vi "ToString.vi"(8 "error in (no error)":errorcluster, 11 "xmlNode in":refnum<class "xmlNode.lvclass">) -> (0 "error out":errorcluster, 2 "xml":string, 3 "xmlNode out":refnum<class "xmlNode.lvclass">)   [LabVIEW 2009, in "Tools.lvlib" / "xml.lvlib" / "xmlNode.lvclass"]
doc: "xml node to xml string (omits the xml title string at the head of an xml document)."
uses:
  xmlNode.lvclass
  xmlNode.lvclass/xmlNode.ctl
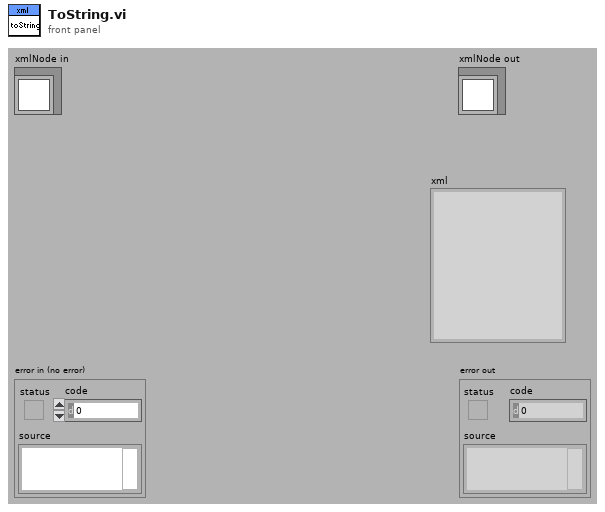
[diagram p1: front panel]
types:
  T1 = cluster{"attribute type":string, "attribute string":string}[]
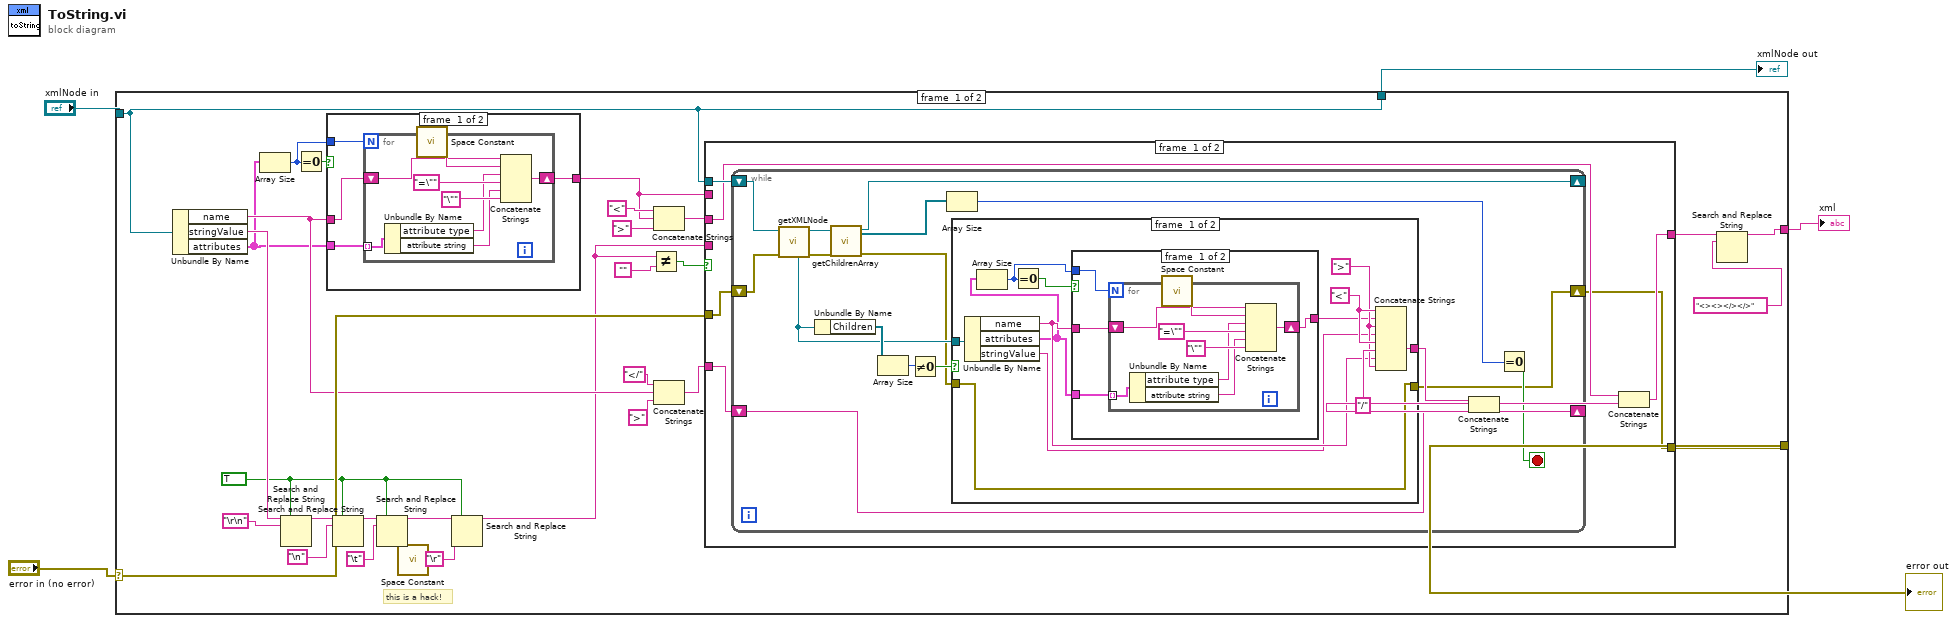
[diagram p0: block diagram]
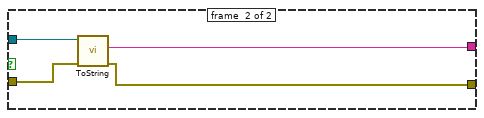
[diagram p4: hidden frame]
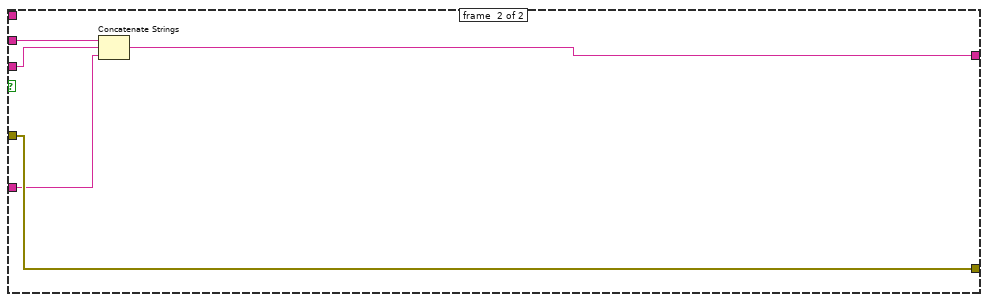
[diagram p5: hidden frame]
diagram:
  n1 = case shown="No Error" "error in (no error)" {
    selector: "error in (no error)" -> [w34 w107]
    tunnel: [w27 w107] -> w4
    tunnel: [w19 w106] -> w2
    tunnel: "xmlNode in" -> [w19 w106]
    tunnel: [w15 _] -> w1
    frame #0 {
      w11 = TRUE
      # "this is a hack!"
      n2 = Unbundle By Name(w19) -> ("name"=w17:string, "stringValue"=w22:string, "attributes"=w6:T1)
      n3 = Array Size(array=w6) -> (size(s)=w7:i32)
      n4 = Search and Replace String(replace all?=w11, input string=w22, search string="\r\n") -> (result string=w26:string)  [unwired: 5 in, 3 out]
      n5 = Equal To 0?(x=w7) -> (x = 0?=w8:bool)
      n6 = case shown="False" w8 {
        tunnel: [w38 w47] -> w18
        tunnel: w17 -> [w37 w47]
        tunnel: w7 -> [w36 _]
        tunnel: w6 -> [w35 _]
        frame #0 {
          n7 = for {
            N: w36 -> [_]
            shift-right: [w43] -> w38
            shift-left: w37 -> [w42]
            tunnel: w35 -> [w41] mode=indexing
            n8 = Unbundle By Name(w41) -> ("attribute type"=w40:string, "attribute string"=w39:string)
            n9 = call <vilib>:"Space Constant.vi"() -> ("String"=w46:string)
            n10 = Concatenate Strings(w42, w46, w40, "=\"", w39, "\"") -> (w43:string)
          }
        }
        frame #1 {
        }
      }
      n11 = Search and Replace String(replace all?=w11, input string=w26, search string="\n") -> (result string=w24:string)  [unwired: 5 in, 3 out]
      n12 = Search and Replace String(replace all?=w11, input string=w24, search string="\t") -> (result string=w9:string)  [unwired: 5 in, 3 out]
      n13 = call <vilib>:"Space Constant.vi"() -> ()  [unwired: 1 out]
      n14 = Search and Replace String(replace all?=w11, input string=w9, search string="\r") -> (result string=w13:string)  [unwired: 5 in, 3 out]
      n15 = Not Equal?(x=w13, y="") -> (x != y?=w12:bool)
      n16 = Concatenate Strings("<", w18, ">") -> (w31:string)
      n17 = Concatenate Strings("</", w17, ">") -> (w28:string)
      n18 = case shown="False" w12 {
        tunnel: w34 -> [w50 w102]
        tunnel: w13 -> [_ w104]
        tunnel: w31 -> [w52 w105]
        tunnel: w18 -> [_ _]
        tunnel: [w51 w103] -> w16
        tunnel: w19 -> [w54 _]
        tunnel: w28 -> [w48 w101]
        tunnel: [w49 w102] -> w27
        frame #0 {
          n19 = while {
            shift-right: [w68] -> _
            shift-left: w54 -> [w65]
            shift-right: [w57] -> w49
            shift-left: w50 -> [w56]
            shift-right: [w58] -> w53
            shift-left: w48 -> [w55]
            stop <- w70 stop-if-true
            n20 = call-dynamic "getXMLNode.vi"("error in (no error)"=w56, "xmlNode in"=w65) -> ("error out"=w66:errorcluster, "xmlNode extracted"=w61:refnum<class "xmlNode.lvclass">, "xmlNode out"=w67:refnum<class "xmlNode.lvclass">)  [unwired: 7 in]
            n21 = Unbundle By Name(w61) -> ("Children"=w64:refnum<class>[])
            n22 = call-dynamic "getChildrenArray.vi"("error in (no error)"=w66, "xmlNode.lvclass in"=w67) -> ("error out"=w60:errorcluster, "Children"=w71:refnum<class "xmlNode.lvclass">[], "xmlNode.lvclass out"=w68:refnum<class "xmlNode.lvclass">)  [unwired: 7 in]
            n23 = Array Size(array=w64) -> (size(s)=w63:i32)
            n24 = Not Equal To 0?(x=w63) -> (x != 0?=w62:bool)
            n25 = Array Size(array=w71) -> (size(s)=w69:i32)
            n26 = case shown="False" w62 {
              tunnel: w61 -> [w83 w100]
              tunnel: w60 -> [w82 w99]
              tunnel: [w78 w98] -> w59
              tunnel: [w82 w97] -> w57
              frame #0 {
                w79 = ">"
                w81 = "<"
                n27 = Unbundle By Name(w83) -> ("name"=w76:string, "attributes"=w73:T1, "stringValue"=w75:string)
                n28 = Array Size(array=w73) -> (size(s)=w72:i32)
                n29 = Equal To 0?(x=w72) -> (x = 0?=w74:bool)
                n30 = case shown="False" w74 {
                  tunnel: [w87 w96] -> w77
                  tunnel: w76 -> [w86 w96]
                  tunnel: w72 -> [w85 _]
                  tunnel: w73 -> [w84 _]
                  frame #0 {
                    n31 = for {
                      N: w85 -> [_]
                      shift-right: [w92] -> w87
                      shift-left: w86 -> [w91]
                      tunnel: w84 -> [w90] mode=indexing
                      n32 = Unbundle By Name(w90) -> ("attribute type"=w89:string, "attribute string"=w88:string)
                      n33 = call <vilib>:"Space Constant.vi"() -> ("String"=w95:string)
                      n34 = Concatenate Strings(w91, w95, w89, "=\"", w88, "\"") -> (w92:string)
                    }
                  }
                  frame #1 {
                  }
                }
                n35 = Concatenate Strings(w81, w77, w79, w75, w81, "/", w76, w79) -> (w78:string)
              }
              frame #1 {
                n36 = call-dynamic "ToString.vi"("error in (no error)"=w99, "xmlNode in"=w100) -> ("error out"=w97:errorcluster, "xml"=w98:string)  [unwired: 7 in, 1 out]
              }
            }
            n37 = Concatenate Strings(w59, w55) -> (w58:string)
            n38 = Equal To 0?(x=w69) -> (x = 0?=w70:bool)
          }
          n39 = Concatenate Strings(w52, w53) -> (w51:string)
        }
        frame #1 {
          n40 = Concatenate Strings(w105, w104, w101) -> (w103:string)
        }
      }
      n41 = Search and Replace String(input string=w16, search string="<><></></>") -> (result string=w15:string)  [unwired: 6 in, 3 out]
    }
    frame #1 {
    }
  }
  "error out" <- w4
  "xmlNode out" <- w2
  "xml" <- w1
